vi "Read Measurement Result (Multiple Points).vi"(7 "Maximum Time (10000 ms)":i32=10000, 8 "error in (no error)":errorcluster, 9 "Data Mode (5: Voltage)":i32(ring)=5 items=["Current", "Resistance", "Source Output Setting", "Status", "Time", "Voltage"], 10 "Channel (0: Channel 1)":i32(ring) items=["Channel 1", "Channel 2"], 11 "VISA resource name":refnum<visa-resource-name>) -> (0 "error out":errorcluster, 2 "Measurement Results":dbl[](array[numeric]), 3 "VISA resource name out":refnum<visa-resource-name>)   [LabVIEW 2026, in "Agilent B2900 Series.lvlib"]
doc: "Reads and fetch the array data in series."
uses:
  Agilent B2900 Series.lvlib
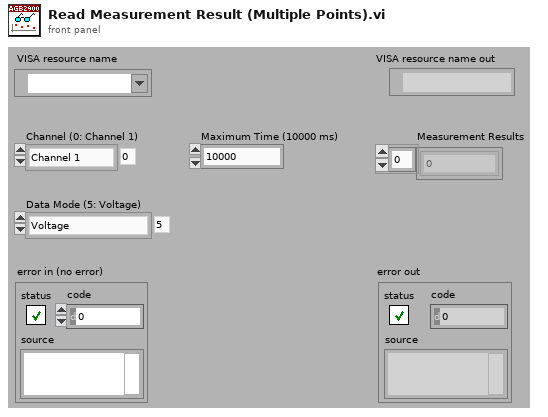
[diagram p1: front panel]
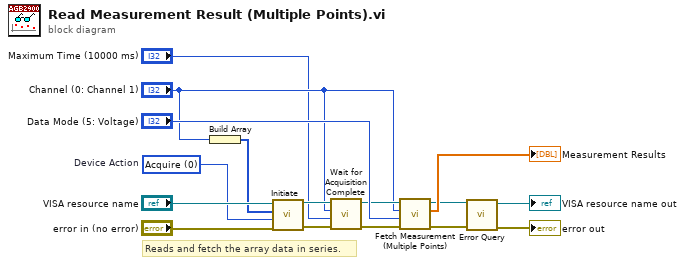
[diagram p0: block diagram]
diagram:
  w8 = 0 items=["Acquire", "Transient", "Both"]  # Device Action
  # "Reads and fetch the array data in series."
  n1 = Build Array("Channel (0: Channel 1)") -> (w10:i32[])
  n2 = call "Initiate.vi"("error in (no error)"="error in (no error)", "Device Action (2: Both)"=w8, "Channel List ({Channel1})"=w10, "VISA resource name"="VISA resource name") -> ("error out"=w7:errorcluster, "VISA resource name out"=w4:refnum<visa-resource-name>)  [unwired: 6 in]
  n3 = call "Wait for Acquisition Complete.vi"("error in (no error)"=w7, "Maximum Time (10000 ms)"="Maximum Time (10000 ms)", "Channel (0: Channel 1)"="Channel (0: Channel 1)", "VISA resource name"=w4) -> ("error out"=w6:errorcluster, "VISA resource name out"=w5:refnum<visa-resource-name>)  [unwired: 6 in]
  n4 = call "Fetch Measurement (Multiple Points).vi"("error in (no error)"=w6, "Data Mode (5: Voltage)"="Data Mode (5: Voltage)", "Channel (0: Channel 1)"="Channel (0: Channel 1)", "VISA resource name"=w5) -> ("error out"=w11:errorcluster, "Measurements"=→"Measurement Results":dbl[], "VISA resource name out"=w12:refnum<visa-resource-name>)  [unwired: 5 in]
  n5 = call "Error Query.vi"("error in (no error)"=w11, "VISA resource name"=w12) -> ("error out"=→"error out":errorcluster, "VISA resource name out"=→"VISA resource name out":refnum<visa-resource-name>)  [unwired: 6 in, 2 out]
